vi "normalise_pulses.vi"(9 "pulses":u32[][](array[numeric]), 10 "stop_read":u32[][](array[numeric]), 11 "detections":u32[](array[numeric])) -> (3 "detections_normalised":dbl[](array[numeric]))   [LabVIEW 2014]
uses:
  <vilib>/Analysis/baseanly.llb/Mean (DBL).vi
  <vilib>/Analysis/NI_AALBase.lvlib
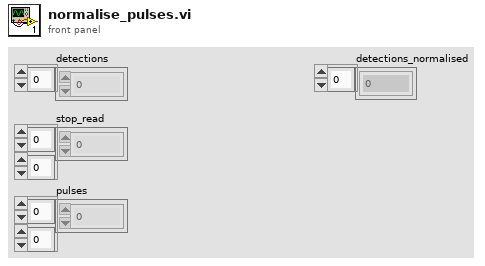
[diagram p1: front panel]
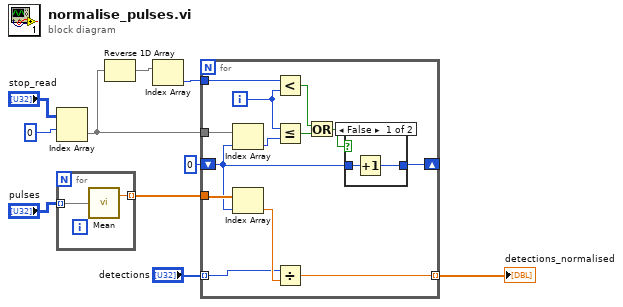
[diagram p0: block diagram]
diagram:
  n1 = Index Array(array="stop_read", index (row)=0) -> (element=w10:u32[])  [unwired: 1 in]
  n2 = for {
    tunnel: "pulses" -> [w12] mode=indexing
    tunnel: [w11] -> w5 mode=indexing
    n3 = call-poly <vilib>:"Mean.vi"("X"=w12) -> ("mean"=w11:dbl)  [unwired: 1 out]
  }
  n4 = Reverse 1D Array(array=w10) -> (reversed array=w9:u32[])
  n5 = Index Array(array=w9) -> (element=w1:u32)  [unwired: 1 in]
  n6 = for {
    tunnel: "detections" -> [w23] mode=indexing
    tunnel: w10 -> [w20]
    tunnel: w5 -> [w25]
    shift-right: [w18] -> _
    shift-left: 0 -> [w19]
    tunnel: [w22] -> w8 mode=indexing
    tunnel: w1 -> [w15]
    i -> [w16]
    n7 = Index Array(array=w20, index=w19) -> (element=w21:u32)
    n8 = Index Array(array=w25, index=w19) -> (element=w24:dbl)
    n9 = Less?(x=w15, y=w16) -> (x < y?=w14:bool)
    n10 = Less Or Equal?(x=w16, y=w21) -> (x <= y?=w13:bool)
    n11 = Divide(x=w23, y=w24) -> (x/y=w22:dbl)
    n12 = Or(x=w14, y=w13) -> (x .or. y?=w17:bool)
    n13 = case shown="False" w17 {
      tunnel: w19 -> [w27 w28]
      tunnel: [w26 w28] -> w18
      frame False {
        n14 = Increment(x=w27) -> (x+1=w26:i32)
      }
      frame True {
      }
    }
  }
  "detections_normalised" <- w8
